vi "Leng Conv.vi"(8 "Unit":bool, 11 "length":string) -> (3 "String":string)   [LabVIEW 2014, in "Programing Logic.lvclass"]
uses:
  Programming Logic/Programing Logic.lvclass
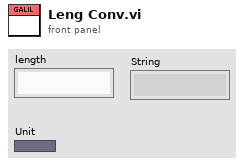
[diagram p1: front panel]
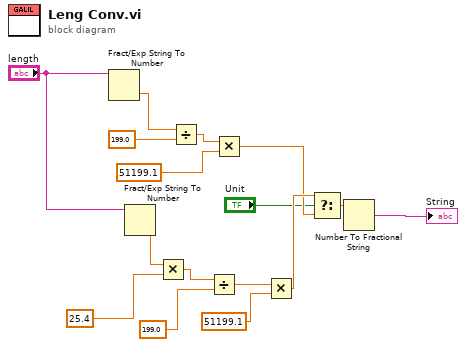
[diagram p0: block diagram]
diagram:
  n1 = Fract/Exp String To Number(string="length") -> (number=w1:dbl)  [unwired: 3 in, 1 out]
  n2 = Fract/Exp String To Number(string="length") -> (number=w6:dbl)  [unwired: 3 in, 1 out]
  n3 = Multiply(x=w6, y=25.4) -> (x*y=w8:dbl)
  n4 = Divide(x=w1, y=199.0) -> (x/y=w3:dbl)
  n5 = Divide(x=w8, y=199.0) -> (x/y=w12:dbl)
  n6 = Multiply(x=w3, y=51199.1) -> (x*y=w15:dbl)
  n7 = Multiply(x=w12, y=51199.1) -> (x*y=w16:dbl)
  n8 = Select(t=w16, s="Unit", f=w15) -> (s? t:f=w10:dbl)
  n9 = Number To Fractional String(number=w10) -> (F-format string=→"String":string)  [unwired: 3 in]
